vi "6509 Pnuematic Outputs.vi"(1 "error in (no error)":errorcluster, 2 "Enable Output":bool, 3 "Enum":T1(ring)) -> (0 "error out":errorcluster)   [LabVIEW 2014]
panel:
  out "data 2":bool[](array[boolean])
  in  "data":bool[](array[boolean])
  # "Pos 4"
  # "pos 5"
  # "Pos 10"
  # "Pos 11"
  # "Pos 12"
  # "Pos 13"
  # "Pos 14"
  # "Pos 15"
  # "Pos 7"
  # "Pos 0"
  # "Pos 1"
  # "Pos 2"
  # "Pos 3"
  # "Pos 6"
  # "Pos 8"
  # "Pos 9"
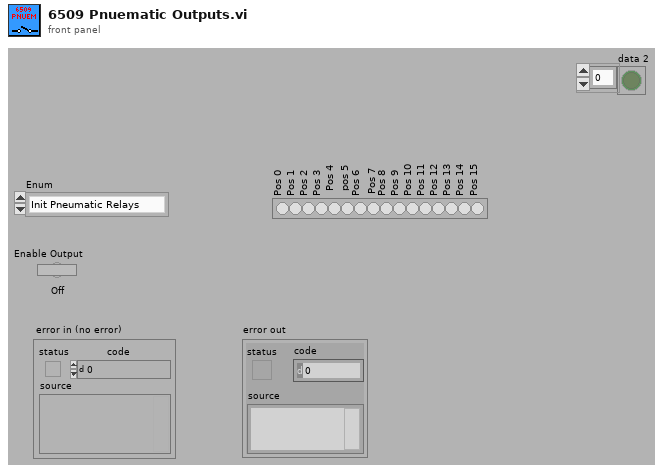
[diagram p1: front panel]
types:
  T1 = enum16{"Init Pneumatic Relays", "Pneumatic_Drive_0", "Pneumatic_Drive_1", "Pneumatic_Drive_2", "Pneumatic_Drive_3", "Pneumatic_Drive_4", "Pneumatic_Drive_5", "Pneumatic_Drive_6", "Pneumatic_Drive_7", "Pneumatic_Drive_8", "Pneumatic_Drive_9", "Pneumatic_Drive_10", "Pneumatic_Drive_11", "Pneumatic_Drive_12", "Pneumatic_Drive_13", "Pneumatic_Drive_14", "Pneumatic_Drive_15"}
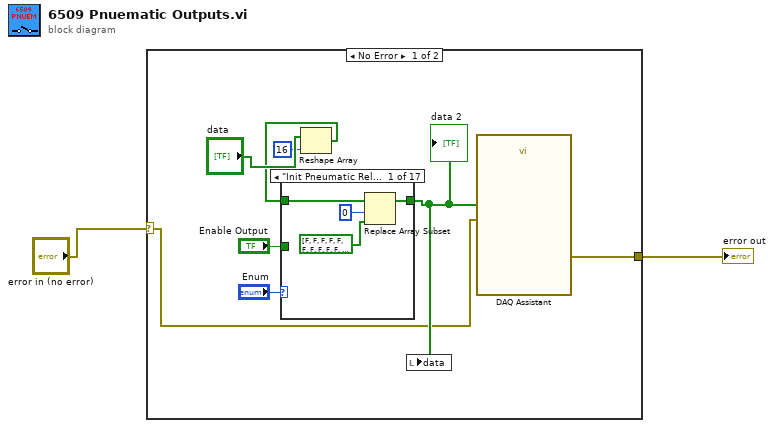
[diagram p0: block diagram]
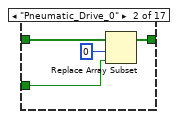
[diagram p2: hidden frame]
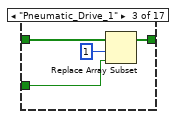
[diagram p3: hidden frame]
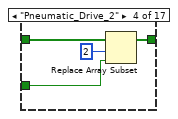
[diagram p4: hidden frame]
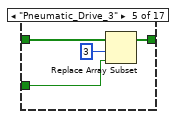
[diagram p5: hidden frame]
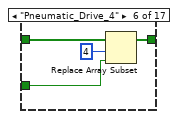
[diagram p6: hidden frame]
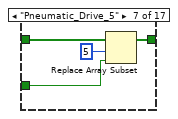
[diagram p7: hidden frame]
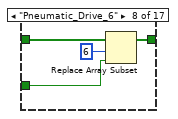
[diagram p8: hidden frame]
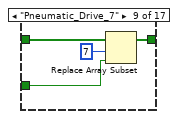
[diagram p9: hidden frame]
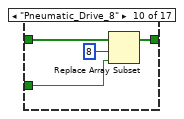
[diagram p10: hidden frame]
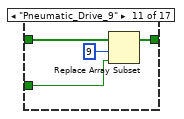
[diagram p11: hidden frame]
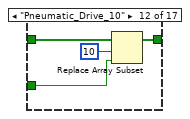
[diagram p12: hidden frame]
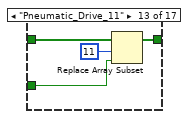
[diagram p13: hidden frame]
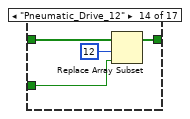
[diagram p14: hidden frame]
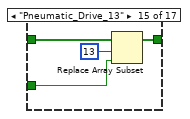
[diagram p15: hidden frame]
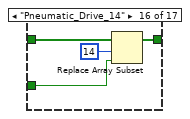
[diagram p16: hidden frame]
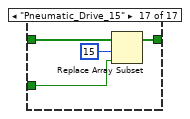
[diagram p17: hidden frame]
diagram:
  n1 = case shown="No Error" "error in (no error)" {
    selector: "error in (no error)" -> [w3 w79]
    tunnel: [w9 w79] -> w2
    frame No Error {
      n2 = Reshape Array("data", 16 ("dimension size")) -> (w5:bool[])
      n3 = case shown="\"Init Pneumatic Relays\", Default" "Enum" {
        tunnel: "Enable Output" -> [_ w18 w20 w24 w28 w32 w36 w40 w44 w48 w52 w56 w60 w64 w68 w72 w76]
        tunnel: w5 -> [w14 w17 w21 w25 w29 w33 w37 w41 w45 w49 w53 w57 w61 w65 w69 w73 w77]
        tunnel: [w12 w15 w19 w23 w27 w31 w35 w39 w43 w47 w51 w55 w59 w63 w67 w71 w75] -> w4
        frame "Init Pneumatic Relays", Default {
          n4 = Replace Array Subset(array=w14, new element=bool[] [FALSE, FALSE, FALSE, FALSE, FALSE, FALSE, FALSE, FALSE, FALSE, FALSE, FALSE, FALSE, FALSE, FALSE, FALSE, FALSE] ("data 2"), index=0) -> (w12:bool[])
        }
        frame "Pneumatic_Drive_0" {
          n5 = Replace Array Subset(array=w17, new element=w18, index=0) -> (w15:bool[])
        }
        frame "Pneumatic_Drive_1" {
          n6 = Replace Array Subset(array=w21, new element=w20, index=1) -> (w19:bool[])
        }
        frame "Pneumatic_Drive_2" {
          n7 = Replace Array Subset(array=w25, new element=w24, index=2) -> (w23:bool[])
        }
        frame "Pneumatic_Drive_3" {
          n8 = Replace Array Subset(array=w29, new element=w28, index=3) -> (w27:bool[])
        }
        frame "Pneumatic_Drive_4" {
          n9 = Replace Array Subset(array=w33, new element=w32, index=4) -> (w31:bool[])
        }
        frame "Pneumatic_Drive_5" {
          n10 = Replace Array Subset(array=w37, new element=w36, index=5) -> (w35:bool[])
        }
        frame "Pneumatic_Drive_6" {
          n11 = Replace Array Subset(array=w41, new element=w40, index=6) -> (w39:bool[])
        }
        frame "Pneumatic_Drive_7" {
          n12 = Replace Array Subset(array=w45, new element=w44, index=7) -> (w43:bool[])
        }
        frame "Pneumatic_Drive_8" {
          n13 = Replace Array Subset(array=w49, new element=w48, index=8) -> (w47:bool[])
        }
        frame "Pneumatic_Drive_9" {
          n14 = Replace Array Subset(array=w53, new element=w52, index=9) -> (w51:bool[])
        }
        frame "Pneumatic_Drive_10" {
          n15 = Replace Array Subset(array=w57, new element=w56, index=10) -> (w55:bool[])
        }
        frame "Pneumatic_Drive_11" {
          n16 = Replace Array Subset(array=w61, new element=w60, index=11) -> (w59:bool[])
        }
        frame "Pneumatic_Drive_12" {
          n17 = Replace Array Subset(array=w65, new element=w64, index=12) -> (w63:bool[])
        }
        frame "Pneumatic_Drive_13" {
          n18 = Replace Array Subset(array=w69, new element=w68, index=13) -> (w67:bool[])
        }
        frame "Pneumatic_Drive_14" {
          n19 = Replace Array Subset(array=w73, new element=w72, index=14) -> (w71:bool[])
        }
        frame "Pneumatic_Drive_15" {
          n20 = Replace Array Subset(array=w77, new element=w76, index=15) -> (w75:bool[])
        }
      }
      "data 2" <- w4
      n21 = local write "data"(w4) -> ()
      n22 = call "DAQ Assistant"("data"=w4, "error in"=w3) -> ("error out"=w9:errorcluster)  [unwired: 16 in, 1 out]
    }
    frame Error {
    }
  }
  "error out" <- w2
